vi "Generate CSM Class API Arguments.vi"(11 "Argument":T1) -> (3 "String":string)   [LabVIEW 2020, in "CSM Mermaid Support.lvlib"]
uses:
  CSM Mermaid Support.lvlib
  <userlib>/_NEVSTOP/Communicable State Machine(CSM)/_csmHelper/Typedef/Def-Argument Info.ctl
  <userlib>/_NEVSTOP/Communicable State Machine(CSM)/Communicable State Machine.lvlib
  <vilib>/Utility/Data Type/NI_Data Type.lvlib
  <userlib>/_NEVSTOP/Communicable State Machine(CSM)/addons/API-String-Arugments-Support/API String Arguments Support.lvlib
  <userlib>/_NEVSTOP/Communicable State Machine(CSM)/_Shared/CSM Shared.lvlib
  <userlib>/_NEVSTOP/Communicable State Machine(CSM)/_csmHelper/CSM-Helper.lvclass
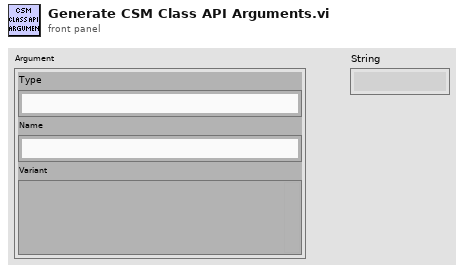
[diagram p1: front panel]
types:
  T1 = typedef "CSM-Helper.lvclass/Def-Argument Info.ctl" = cluster{"Type":string, "Name":string, "Variant":variant}
  T2 = typedef "NI_Data Type.lvlib/Data Type.ctl" = enum8{"Invalid Type", "Void", "I8", "I16", "I32", "I64", "U8", "U16", "U32", "U64", "Single Float", "Double Float", "Extended Float", "Single Complex", "Double Complex", "Extended Complex", "Enum U8", "Enum U16", "Enum U32", "Enum U64", "Single Float With Unit", "Double Float With Unit", "Extended Float With Unit", "Single Complex with Unit", "Double Complex with Unit", "Extended Complex with Unit", "Boolean", "String", "Path", "Picture", "Tag", "Array", "Cluster", "Variant", "LV Variant", "Waveform", "Timestamp", "Digital Waveform", "Digital Data", "ExpressData", "Refnum", "External Data", "VI", "Poly VI", "LabVIEW Class Instance", "Fixed Point", "Set Collection", "Map Collection"}
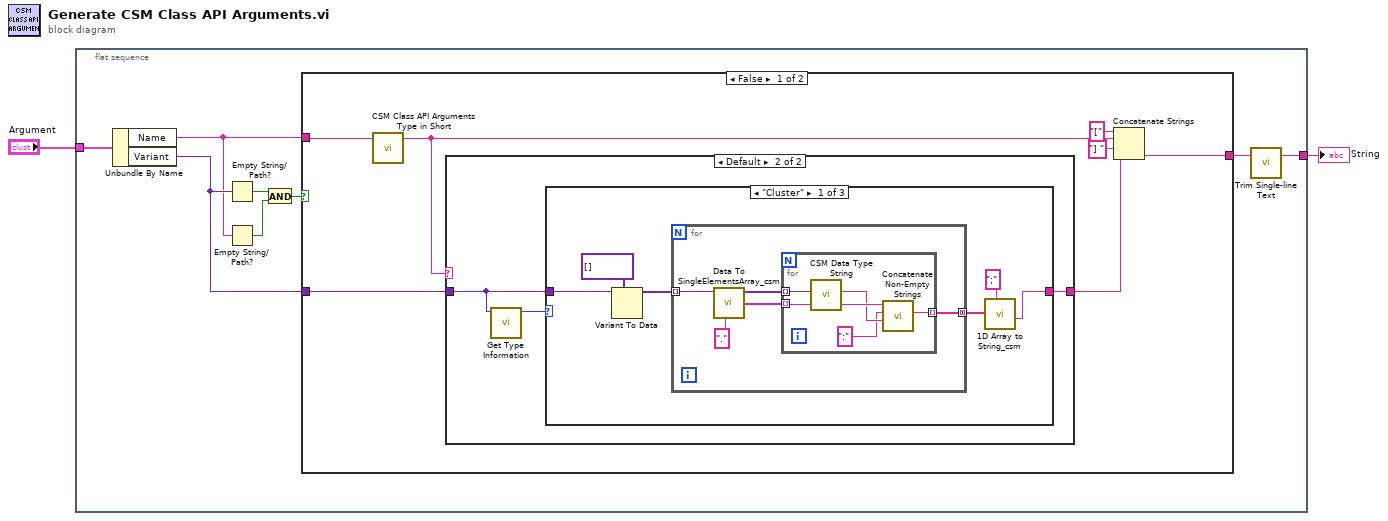
[diagram p0: block diagram]
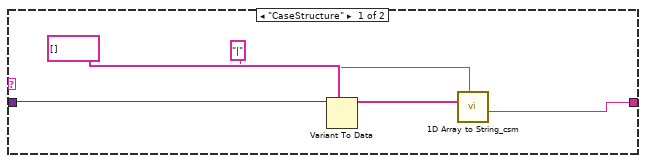
[diagram p2: hidden frame]
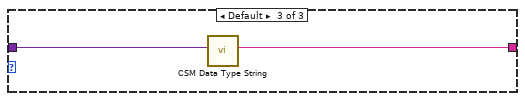
[diagram p4: hidden frame]
diagram:
  n1 = flat-sequence {
    tunnel: [w3] -> w2
    tunnel: "Argument" -> [w7]
    frame #0 {
      n2 = Unbundle By Name(w7) -> ("Name"=w4:string, "Variant"=w9:variant)
      n3 = Empty String/Path?(string/path=w9) -> (empty?=w10:bool)
      n4 = Empty String/Path?(string/path=w4) -> (empty?=w5:bool)
      n5 = And(x=w10, y=w5) -> (x .and. y?=w6:bool)
      n6 = case shown="False" w6 {
        tunnel: [w15 _] -> w8
        tunnel: w9 -> [w16 _]
        tunnel: w4 -> [w12 _]
        frame False {
          n7 = call "CSM Class API Arguments Type in Short.vi"("String"=w12) -> ("s? t:f"=w11:string)  [unwired: 10 in]
          n8 = case shown="Default" w11 {
            tunnel: [w18 w25] -> w17
            tunnel: w16 -> [w22 w24]
            frame "CaseStructure" {
              n9 = Variant To Data(type=string[] [] ("string"), Variant=w22) -> (data=w20:string[])  [unwired: 1 in, 1 out]
              n10 = call <userlib>:"1D Array to String_csm.vi"("delimiter (Tab)"="|" ("string"), "Array of Strings"=w20) -> ("delimited string"=w18:string)  [unwired: 9 in]
            }
            frame Default {
              n11 = call <vilib>:"Get Type Information.vi"("variant"=w24) -> ("type"=w23:T2)  [unwired: 6 in, 4 out]
              n12 = case shown="\"Cluster\"" w23 {
                tunnel: [w29 _ w43] -> w25
                tunnel: w24 -> [w27 _ w42]
                frame "Cluster" {
                  n13 = Variant To Data(type=variant[] [] ("Array"), Variant=w27) -> (data=w26:variant[])  [unwired: 1 in, 1 out]
                  n14 = for {
                    tunnel: [w34] -> w31 mode=concatenating
                    tunnel: w26 -> [w32] mode=indexing
                    n15 = call <userlib>:"Data To SingleElementsArray_csm.vi"("Seperator(/)"=".", "Cluster"=w32) -> ("Full NameList"=w35:string[], "DataElementArray"=w36:variant[])  [unwired: 7 in, 1 out]
                    n16 = for {
                      tunnel: w36 -> [w41] mode=indexing
                      tunnel: w35 -> [w40] mode=indexing
                      tunnel: [w39] -> w34 mode=indexing
                      n17 = call <userlib>:"CSM Data Type String.vi"("Data"=w41) -> ("Data Type String"=w38:string)  [unwired: 10 in]
                      n18 = call <userlib>:"Concatenate Non-Empty Strings.vi"("String2"=w38, "Seperator(Carriage Return)"=":" ("seperator(:)"), "String1"=w40) -> ("Result String"=w39:string)  [unwired: 5 in]
                    }
                  }
                  n19 = call <userlib>:"1D Array to String_csm.vi"("delimiter (Tab)"=";", "Array of Strings"=w31) -> ("delimited string"=w29:string)  [unwired: 9 in]
                }
                frame "Void" {
                }
                frame Default {
                  n20 = call <userlib>:"CSM Data Type String.vi"("Data"=w42) -> ("Data Type String"=w43:string)  [unwired: 10 in]
                }
              }
            }
          }
          n21 = Concatenate Strings("[" ("string"), w11, "] " ("string"), w17) -> (w15:string)
        }
        frame True {
        }
      }
      n22 = call <userlib>:"Trim Single-line Text.vi"("single-line text"=w8) -> ("trimed text"=w3:string)  [unwired: 2 in]
    }
  }
  "String" <- w2
